vi "PLCModbusExecute.vi"(8 "error in (no error)":errorcluster) -> (0 "error IO":errorcluster)   [LabVIEW 2019]
uses:
  Subvi/RobotControlQueueIn.vi
  LLB/Commonly VI/Main Glb.vi
  <vilib>/NI/Modbus Library/API/Wrapper/Create TCP Master.vi
  <vilib>/NI/Modbus Library/API/Master/Modbus Master.lvclass
  <vilib>/NI/Modbus Library/API/Wrapper/API Main.lvlib
  LLB/Commonly VI.lvlib
panel:
  out "string 2":string
  out "Holding Registers":u16[](array[numeric])
  in  "Boolean":bool=TRUE
  out "Holding Registers 3":u16[](array[numeric])
  out "Sat Coils":bool[](array[boolean])
  out "Holding Registers 2":u16[](array[numeric])
  in  "Coils":bool[](array[boolean])=[FALSE, FALSE, FALSE, FALSE, FALSE, FALSE, FALSE, FALSE]
  out "string":string
  out "Discrete Inputs":bool[](array[boolean])
  in  "stop":bool
  out "Input Registers":u16[](array[numeric])
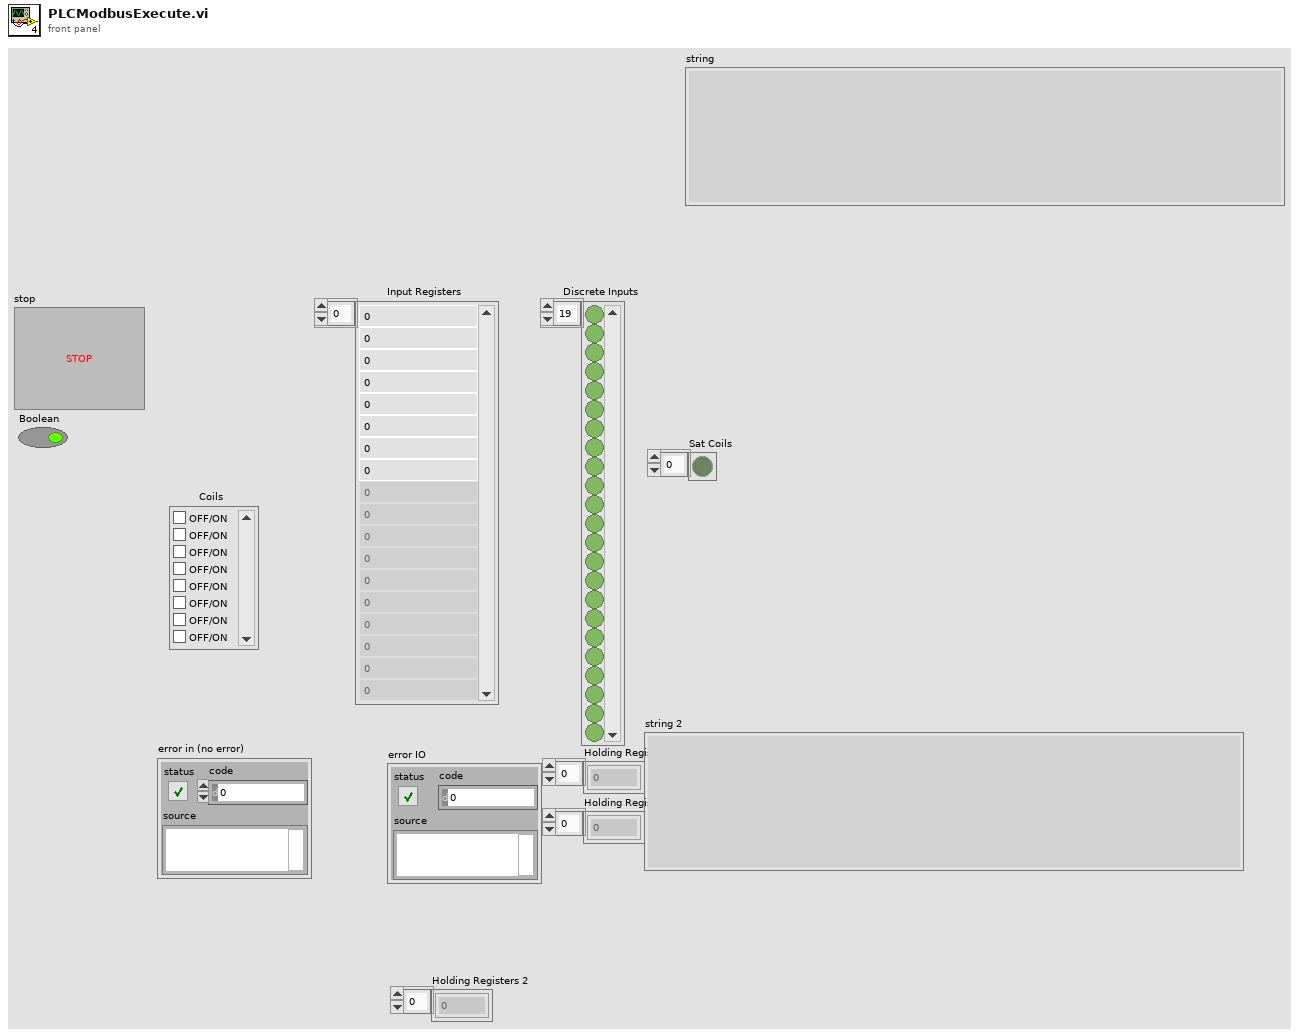
[diagram p1: front panel]
types:
  T1 = cluster{"starting address":u16, "number of inputs":u16, "Sat Coils":bool[], "Holding Registers":u16[]}
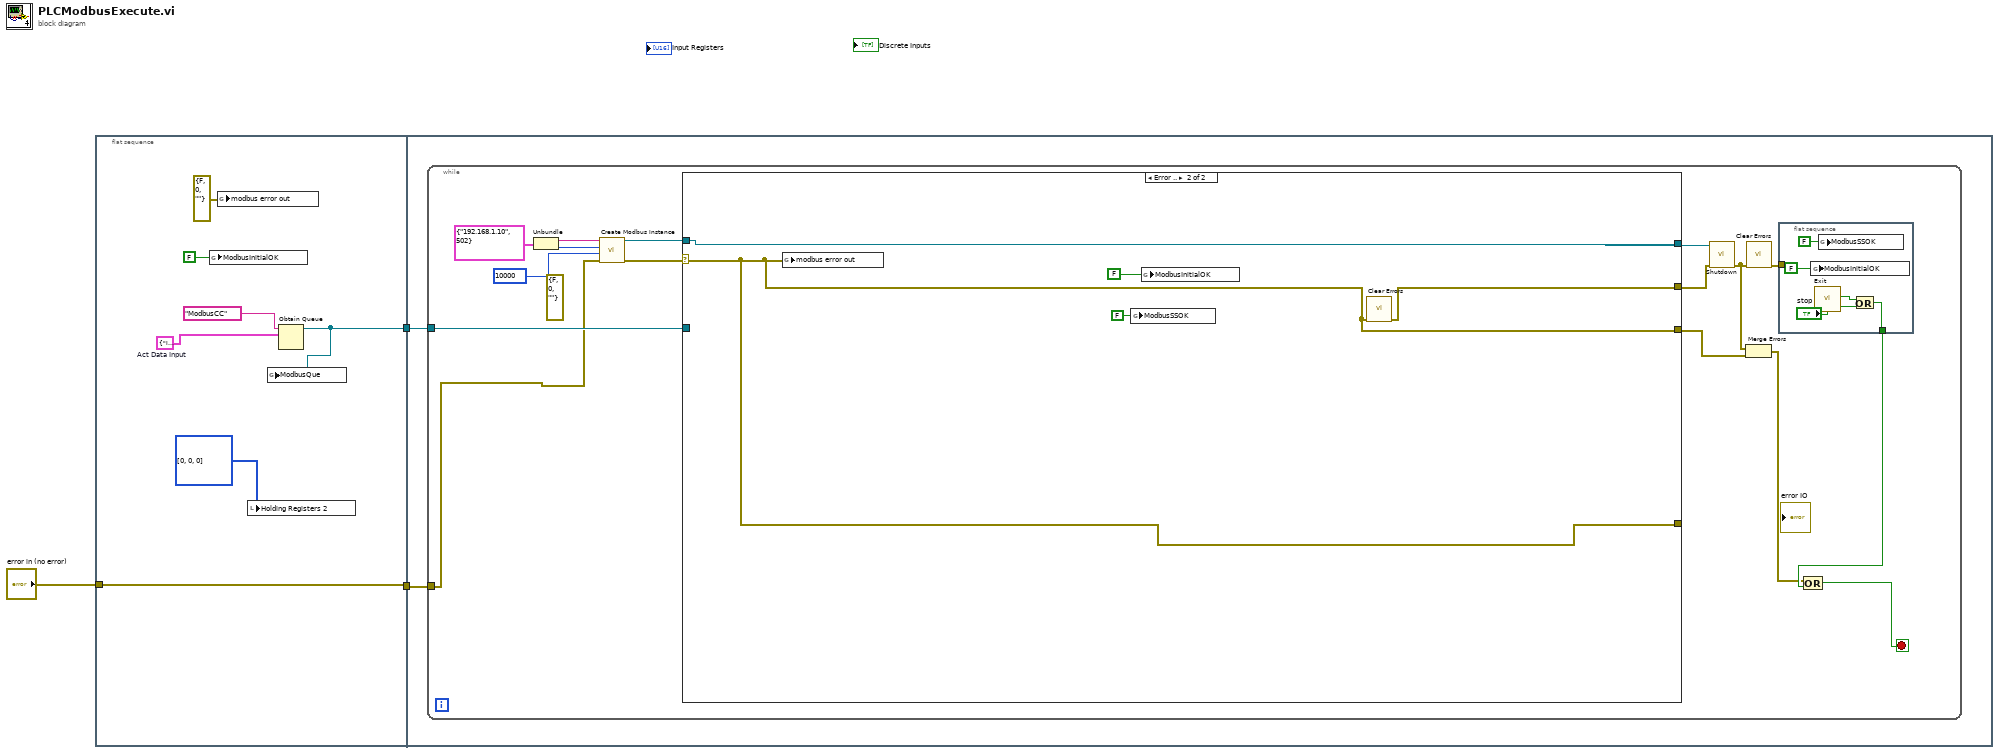
[diagram p0: block diagram]
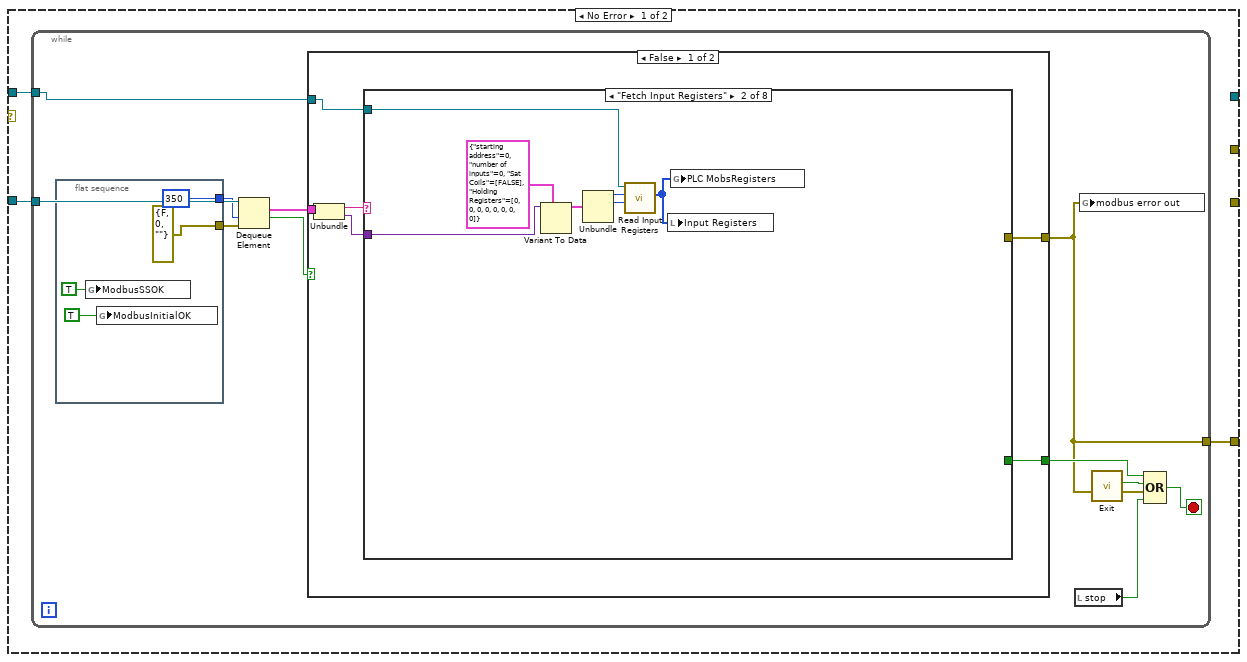
[diagram p2: hidden frame]
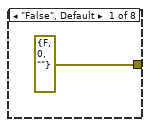
[diagram p3: hidden frame]
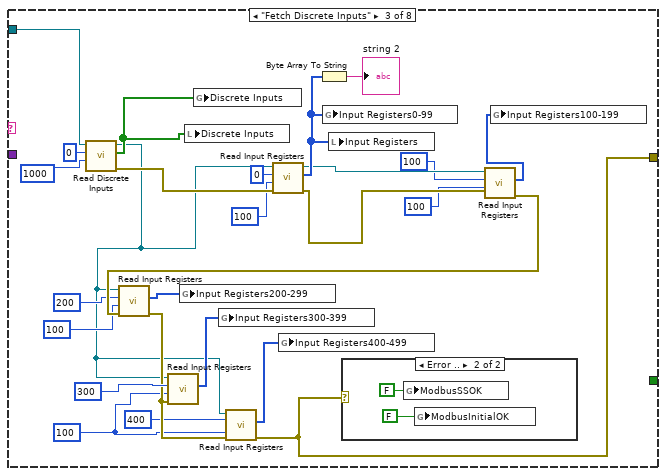
[diagram p4: hidden frame]
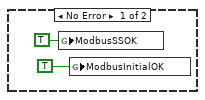
[diagram p5: hidden frame]
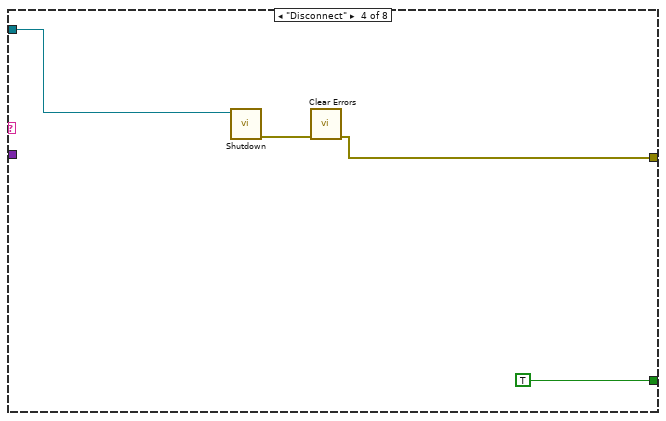
[diagram p6: hidden frame]
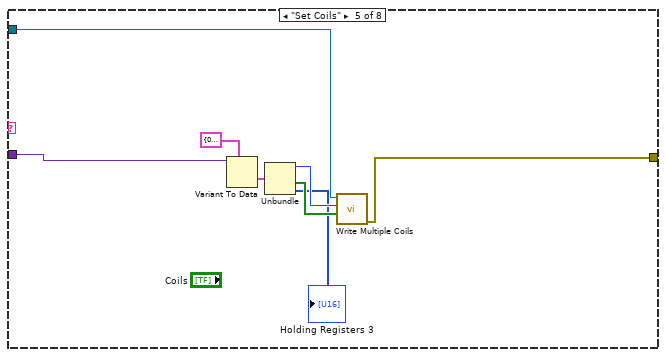
[diagram p7: hidden frame]
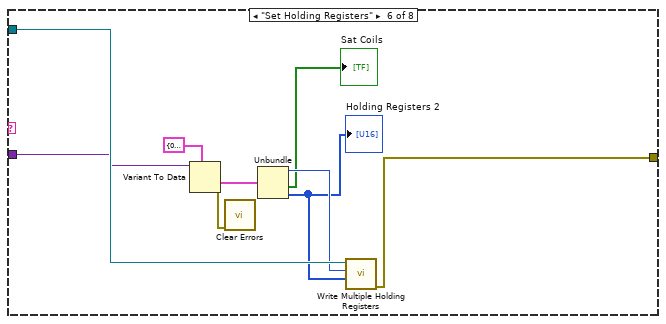
[diagram p8: hidden frame]
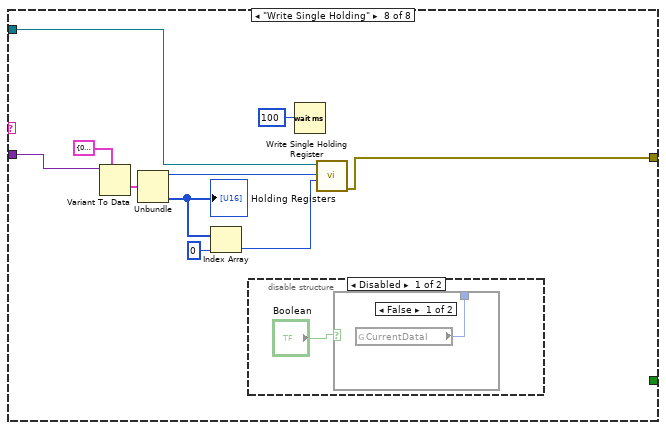
[diagram p10: hidden frame]
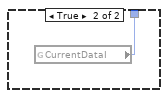
[diagram p11: hidden frame]
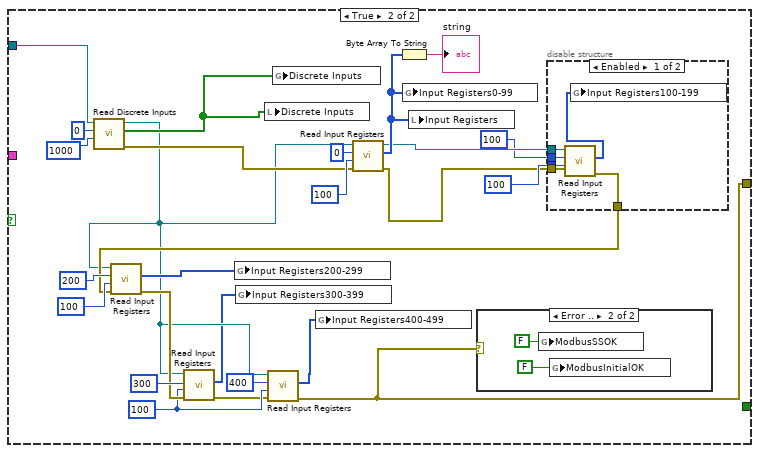
[diagram p13: hidden frame]
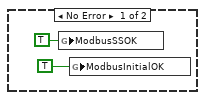
[diagram p15: hidden frame]
diagram:
  n1 = flat-sequence {
    tunnel: [w7] -> w3
    tunnel: "error in (no error)" -> [w5]
    tunnel: [w5] -> w1
    tunnel: w3 -> [w12]
    tunnel: w1 -> [w11]
    frame #0 {
      w9 = cluster{"Act":string, "Data":variant} {"Act"="Init", "Data"=variant}  # Act Data Input
      n2 = global write "Main Glb.vi" "ModbusInitialOK"(FALSE) -> ()
      n3 = global write "Main Glb.vi" "modbus error out"(errorcluster {"status"=FALSE, "code"=0, "source"=""} ("modbus error out")) -> ()
      n4 = local write "Holding Registers 2"(u16[] [0, 0, 0] ("Holding Registers 2")) -> ()
      n5 = Obtain Queue(name (unnamed)="ModbusCC", element data type=w9) -> (queue out=w7:refnum<queue>)  [unwired: 3 in, 2 out]
      n6 = global write "RobotControlQueueIn.vi" "ModbusQue"(w7) -> ()
    }
    frame #1 {
      n7 = while {
        tunnel: w12 -> [w23]
        tunnel: w11 -> [w16]
        stop <- w18 stop-if-true
        (unwired) errorcluster {"status"=FALSE, "code"=0, "source"=""} ("error in")
        n8 = Unbundle(cluster{"Slave Address":string, "Port":u16} {"Slave Address"="192.168.1.10", "Port"=502} ("Slave")) -> ("Slave Address"=w27:string, "Port"=w26:u16)
        n9 = call-poly <vilib>:"Create Modbus Instance.vi"("error in"=w16, "connect timeout ms"=10000, "port (502)"=w26, "address"=w27) -> ("error out"=w25:errorcluster, "TCP master instance"=w24:refnum<class "Modbus Master.lvclass">)  [unwired: 6 in]
        n10 = case shown="Error .." w25 {
          selector: w25 -> [_ w168]
          tunnel: w24 -> [w35 w169]
          tunnel: w23 -> [w36 _]
          tunnel: [_ w169] -> w22
          tunnel: [w34 w168] -> _
          tunnel: [_ w170] -> w17
          tunnel: [_ w168] -> w14
          frame No Error {
            n11 = while {
              tunnel: w36 -> [w47]
              tunnel: w35 -> [w37]
              tunnel: [w40] -> w34
              stop <- w38 stop-if-true
              n12 = flat-sequence {
                tunnel: [errorcluster {"status"=FALSE, "code"=0, "source"=""} ("error constant")] -> w45
                tunnel: [350 ("timeout in ms (-1)")] -> w44
                frame #0 {
                  n13 = global write "Main Glb.vi" "ModbusSSOK"(TRUE ("ModbusSSOK")) -> ()
                  n14 = global write "Main Glb.vi" "ModbusInitialOK"(TRUE) -> ()
                }
              }
              n15 = Dequeue Element(queue=w47, timeout in ms (-1)=w44, error in (no error)=w45) -> (element=w46:cluster{"Act":string, "Data":variant}, timed out?=w43:bool)  [unwired: 2 out]
              n16 = case shown="False" w43 {
                tunnel: w46 -> [w53 _]
                tunnel: [w49 w128] -> w40
                tunnel: w37 -> [w48 w147]
                tunnel: [w50 _] -> w41
                frame False {
                  n17 = Unbundle(w53) -> ("Act"=w52:string, "Data"=w51:variant)
                  n18 = case shown="\"Fetch Input Registers\"" w52 {
                    tunnel: w51 -> [_ w57 _ _ w99 w108 _ w119]
                    tunnel: [_ _ _ TRUE _ _ _ _] -> w50
                    tunnel: [errorcluster {"status"=FALSE, "code"=0, "source"=""} ("error out") _ w63 w93 w98 w112 _ w118] -> w49
                    tunnel: w48 -> [_ w55 w70 w92 w97 w111 _ w122]
                    frame "False", Default {
                    }
                    frame "Fetch Input Registers" {
                      n19 = Variant To Data(type=T1 {"starting address"=0, "number of inputs"=0, "Sat Coils"=[FALSE], "Holding Registers"=[0, 0, 0, 0, 0, 0, 0, 0]} ("output cluster 2"), Variant=w57) -> (data=w61:T1)  [unwired: 1 in, 1 out]
                      n20 = Unbundle(w61) -> ("starting address"=w60:u16, "number of inputs"=w56:u16)  [unwired: 2 out]
                      n21 = call-dynamic "Read Input Registers.vi"("number of inputs"=w56, "starting address"=w60, "Modbus master in"=w55) -> ("register values"=w59:u16[])  [unwired: 6 in, 2 out]
                      n22 = local write "Input Registers"(w59) -> ()
                      n23 = global write "Main Glb.vi" "PLC MobsRegisters"(w59) -> ()
                    }
                    frame "Fetch Discrete Inputs" {
                      w65 = u16 100 ("starting address")
                      n24 = call-dynamic "Read Discrete Inputs.vi"("number of inputs"=u16 1000 ("starting address"), "starting address"=u16 0, "Modbus master in"=w70) -> ("error out"=w84:errorcluster, "discrete inputs"=w87:bool[], "Modbus master out"=w64:refnum<class "Modbus Master.lvclass">)  [unwired: 6 in]
                      n25 = local write "Discrete Inputs"(w87) -> ()
                      n26 = global write "Main Glb.vi" "Discrete Inputs"(w87) -> ()
                      n27 = call-dynamic "Read Input Registers.vi"("error in"=w84, "number of inputs"=u16 100 ("starting address"), "starting address"=u16 0, "Modbus master in"=w64) -> ("error out"=w82:errorcluster, "register values"=w86:u16[], "Modbus master out"=w83:refnum<class "Modbus Master.lvclass">)  [unwired: 5 in]
                      n28 = Byte Array To String(unsigned byte array=w86) -> (string=→"string 2":string)
                      n29 = global write "Main Glb.vi" "Input Registers0-99"(w86) -> ()
                      n30 = local write "Input Registers"(w86) -> ()
                      n31 = call-dynamic "Read Input Registers.vi"("error in"=w82, "number of inputs"=u16 100 ("starting address"), "starting address"=u16 100, "Modbus master in"=w83) -> ("error out"=w81:errorcluster, "register values"=w71:u16[])  [unwired: 5 in, 1 out]
                      n32 = call-dynamic "Read Input Registers.vi"("error in"=w81, "number of inputs"=u16 100 ("starting address"), "starting address"=u16 200, "Modbus master in"=w64) -> ("error out"=w67:errorcluster, "register values"=w80:u16[])  [unwired: 5 in, 1 out]
                      n33 = call-dynamic "Read Input Registers.vi"("error in"=w67, "number of inputs"=w65, "starting address"=u16 300, "Modbus master in"=w64) -> ("register values"=w68:u16[])  [unwired: 5 in, 2 out]
                      n34 = global write "Main Glb.vi" "Input Registers200-299"(w80) -> ()
                      n35 = global write "Main Glb.vi" "Input Registers300-399"(w68) -> ()
                      n36 = call-dynamic "Read Input Registers.vi"("error in"=w67, "number of inputs"=w65, "starting address"=u16 400, "Modbus master in"=w64) -> ("error out"=w63:errorcluster, "register values"=w62:u16[])  [unwired: 5 in, 1 out]
                      n37 = global write "Main Glb.vi" "Input Registers400-499"(w62) -> ()
                      n38 = case shown="Error .." w63 {
                        frame No Error {
                          n39 = global write "Main Glb.vi" "ModbusSSOK"(TRUE ("ModbusSSOK")) -> ()
                          n40 = global write "Main Glb.vi" "ModbusInitialOK"(TRUE) -> ()
                        }
                        frame Error {
                          n41 = global write "Main Glb.vi" "ModbusSSOK"(FALSE ("ModbusSSOK")) -> ()
                          n42 = global write "Main Glb.vi" "ModbusInitialOK"(FALSE) -> ()
                        }
                      }
                      n43 = global write "Main Glb.vi" "Input Registers100-199"(w71) -> ()
                    }
                    frame "Disconnect" {
                      n44 = call-dynamic "Shutdown.vi"("Modbus master in"=w92) -> ("error out"=w94:errorcluster)  [unwired: 10 in]
                      n45 = call <vilib>:"Clear Errors.vi"("error in (no error)"=w94) -> ("error out"=w93:errorcluster)  [unwired: 5 in, 1 out]
                    }
                    frame "Set Coils" {
                      n46 = Variant To Data(type=T1 {"starting address"=0, "number of inputs"=0, "Sat Coils"=[FALSE], "Holding Registers"=[0, 0, 0, 0, 0, 0, 0, 0]} ("output cluster 2"), Variant=w99) -> (data=w100:T1)  [unwired: 1 in, 1 out]
                      n47 = Unbundle(w100) -> ("starting address"=w101:u16, "Sat Coils"=w102:bool[], "Holding Registers"=→"Holding Registers 3":u16[])  [unwired: 1 out]
                      n48 = call-dynamic "Write Multiple Coils.vi"("coils to write"=w102, "starting address"=w101, "Modbus master in"=w97) -> ("error out"=w98:errorcluster)  [unwired: 7 in, 1 out]
                    }
                    frame "Set Holding Registers" {
                      n49 = Variant To Data(type=T1 {"starting address"=0, "number of inputs"=0, "Sat Coils"=[FALSE], "Holding Registers"=[0, 0, 0, 0, 0, 0, 0, 0]} ("output cluster 2"), Variant=w108) -> (data=w110:T1, error out=w107:errorcluster)  [unwired: 1 in]
                      n50 = call <vilib>:"Clear Errors.vi"("error in (no error)"=w107) -> ()  [unwired: 5 in, 2 out]
                      n51 = Unbundle(w110) -> ("starting address"=w106:u16, "Sat Coils"=→"Sat Coils":bool[], "Holding Registers"=w104:u16[])  [unwired: 1 out]
                      "Holding Registers 2" <- w104
                      n52 = call-dynamic "Write Multiple Holding Registers.vi"("registers to write"=w104, "starting address"=w106, "Modbus master in"=w111) -> ("error out"=w112:errorcluster)  [unwired: 7 in, 1 out]
                    }
                    frame "Connect" {
                    }
                    frame "Write Single Holding" {
                      n53 = Variant To Data(type=T1 {"starting address"=0, "number of inputs"=0, "Sat Coils"=[FALSE], "Holding Registers"=[0, 0, 0, 0, 0, 0, 0, 0]} ("output cluster 2"), Variant=w119) -> (data=w121:T1)  [unwired: 1 in, 1 out]
                      n54 = Unbundle(w121) -> ("starting address"=w117:u16, "Holding Registers"=w115:u16[])  [unwired: 2 out]
                      "Holding Registers" <- w115
                      n55 = Index Array(array=w115, index=0) -> (element=w113:u16)
                      n56 = disable-structure shown="Disabled" {
                        frame Disabled {
                          n57 = case shown="False" "Boolean" {
                            tunnel: [w124 w125] -> _
                            frame False {
                              n58 = global read "Main Glb.vi" "CurrentDataI"() -> (w124:i32)
                            }
                            frame True {
                              n59 = global read "Main Glb.vi" "CurrentDataI"() -> (w125:i32)
                            }
                          }
                        }
                        frame Enabled {
                        }
                      }
                      n60 = Wait (ms)(milliseconds to wait=100) -> ()  [unwired: 1 out]
                      n61 = call-dynamic "Write Single Holding Register.vi"("register to write"=w113, "address"=w117, "Modbus master in"=w122) -> ("error out"=w118:errorcluster)  [unwired: 7 in, 1 out]
                    }
                  }
                }
                frame True {
                  w130 = u16 100 ("starting address")
                  n62 = call-dynamic "Read Discrete Inputs.vi"("number of inputs"=u16 1000 ("starting address"), "starting address"=u16 0, "Modbus master in"=w147) -> ("error out"=w143:errorcluster, "discrete inputs"=w151:bool[], "Modbus master out"=w132:refnum<class "Modbus Master.lvclass">)  [unwired: 6 in]
                  n63 = local write "Discrete Inputs"(w151) -> ()
                  n64 = global write "Main Glb.vi" "Discrete Inputs"(w151) -> ()
                  n65 = call-dynamic "Read Input Registers.vi"("error in"=w143, "number of inputs"=u16 100 ("starting address"), "starting address"=u16 0, "Modbus master in"=w132) -> ("error out"=w139:errorcluster, "register values"=w145:u16[], "Modbus master out"=w142:refnum<class "Modbus Master.lvclass">)  [unwired: 5 in]
                  n66 = Byte Array To String(unsigned byte array=w145) -> (string=→"string":string)
                  n67 = global write "Main Glb.vi" "Input Registers0-99"(w145) -> ()
                  n68 = local write "Input Registers"(w145) -> ()
                  n69 = disable-structure shown="Enabled" {
                    disable-tunnel: w142 -> [w157 _]
                    disable-tunnel: u16 100 ("starting address") -> [w156 _]
                    disable-tunnel: u16 100 ("starting address") -> [w155 _]
                    disable-tunnel: w139 -> [w153 w158]
                    disable-tunnel: [w152 w158] -> w136
                    frame Enabled {
                      n70 = call-dynamic "Read Input Registers.vi"("error in"=w153, "number of inputs"=w155, "starting address"=w156, "Modbus master in"=w157) -> ("error out"=w152:errorcluster, "register values"=w154:u16[])  [unwired: 5 in, 1 out]
                      n71 = global write "Main Glb.vi" "Input Registers100-199"(w154) -> ()
                    }
                    frame Disabled {
                    }
                  }
                  n72 = call-dynamic "Read Input Registers.vi"("error in"=w136, "number of inputs"=u16 100 ("starting address"), "starting address"=u16 200, "Modbus master in"=w132) -> ("error out"=w133:errorcluster, "register values"=w135:u16[])  [unwired: 5 in, 1 out]
                  n73 = call-dynamic "Read Input Registers.vi"("error in"=w133, "number of inputs"=w130, "starting address"=u16 300, "Modbus master in"=w132) -> ("error out"=w129:errorcluster, "register values"=w127:u16[])  [unwired: 5 in, 1 out]
                  n74 = global write "Main Glb.vi" "Input Registers200-299"(w135) -> ()
                  n75 = global write "Main Glb.vi" "Input Registers300-399"(w127) -> ()
                  n76 = call-dynamic "Read Input Registers.vi"("error in"=w129, "number of inputs"=w130, "starting address"=u16 400, "Modbus master in"=w132) -> ("error out"=w128:errorcluster, "register values"=w126:u16[])  [unwired: 5 in, 1 out]
                  n77 = global write "Main Glb.vi" "Input Registers400-499"(w126) -> ()
                  n78 = case shown="Error .." w128 {
                    frame No Error {
                      n79 = global write "Main Glb.vi" "ModbusSSOK"(TRUE ("ModbusSSOK")) -> ()
                      n80 = global write "Main Glb.vi" "ModbusInitialOK"(TRUE) -> ()
                    }
                    frame Error {
                      n81 = global write "Main Glb.vi" "ModbusSSOK"(FALSE ("ModbusSSOK")) -> ()
                      n82 = global write "Main Glb.vi" "ModbusInitialOK"(FALSE) -> ()
                    }
                  }
                }
              }
              n83 = local read "stop"() -> (w39:bool)
              n84 = global write "Main Glb.vi" "modbus error out"(w40) -> ()
              n85 = call "Exit.vi"() -> ("ExitOut"=w42:bool)  [unwired: 11 in]
              n86 = Compound Arithmetic op=OR(w41, w42, w40, w39) -> (w38:bool)
            }
          }
          frame Error {
            n87 = global write "Main Glb.vi" "modbus error out"(w168) -> ()
            n88 = global write "Main Glb.vi" "ModbusSSOK"(FALSE ("ModbusSSOK")) -> ()
            n89 = global write "Main Glb.vi" "ModbusInitialOK"(FALSE) -> ()
            n90 = call <vilib>:"Clear Errors.vi"("error in (no error)"=w168) -> ("error out"=w170:errorcluster)  [unwired: 5 in, 1 out]
          }
        }
        n91 = call-dynamic "Shutdown.vi"("error in"=w17, "Modbus master in"=w22) -> ("error out"=w15:errorcluster)  [unwired: 9 in]
        n92 = Merge Errors(w15, w14) -> (w13:errorcluster)
        n93 = call <vilib>:"Clear Errors.vi"("error in (no error)"=w15) -> ("error out"=w20:errorcluster)  [unwired: 5 in, 1 out]
        n94 = flat-sequence {
          tunnel: w20 -> [_]
          tunnel: [w30] -> w19
          frame #0 {
            n95 = global write "Main Glb.vi" "ModbusInitialOK"(FALSE) -> ()
            n96 = call "Exit.vi"() -> ("ExitOut"=w31:bool)  [unwired: 11 in]
            n97 = global write "Main Glb.vi" "ModbusSSOK"(FALSE ("ModbusSSOK")) -> ()
            n98 = Or(x=w31, y="stop") -> (x .or. y?=w30:bool)
          }
        }
        n99 = Compound Arithmetic op=OR(w13, w19) -> (w18:bool)
      }
    }
  }
